vi "initialize_constants.vi"(8 "error in (no error)":errorcluster) -> (0 "error out":errorcluster)   [LabVIEW 2021]
uses:
  Constants.vi
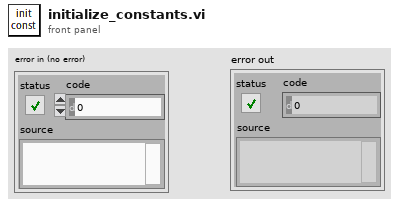
[diagram p1: front panel]
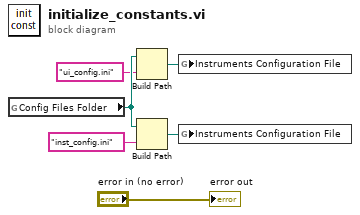
[diagram p0: block diagram]
diagram:
  n1 = global read "Constants.vi" "Config Files Folder"() -> (w3:path)
  n2 = Build Path(base path=w3, name or relative path="ui_config.ini") -> (appended path=w4:path)
  n3 = Build Path(base path=w3, name or relative path="inst_config.ini") -> (appended path=w5:path)
  n4 = global write "Constants.vi" "Instruments Configuration File"(w4) -> ()
  n5 = global write "Constants.vi" "Instruments Configuration File"(w5) -> ()
  "error out" <- "error in (no error)"
